vi "cw_2.vi"() -> ()   [LabVIEW 2022 SP3]
panel:
  out "sin(x)":dbl
  in  "dx":dbl
  out "Waveform Chart":dbl(graph)
  in  "stop":bool
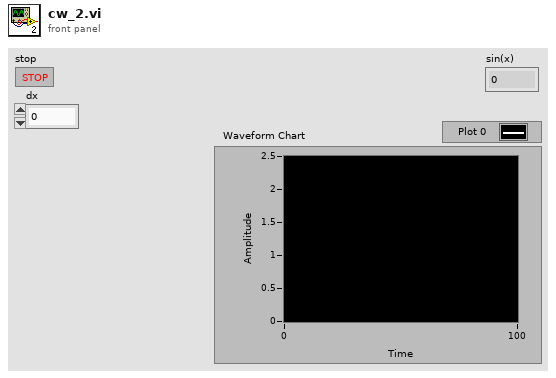
[diagram p1: front panel]
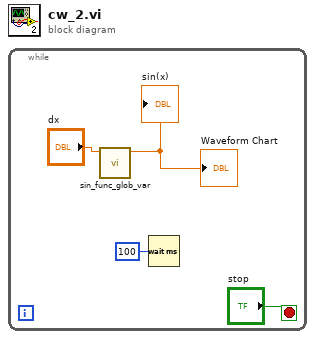
[diagram p0: block diagram]
diagram:
  n1 = while {
    stop <- "stop" stop-if-true
    n2 = call "sin_func_glob_var.vi"("dx"="dx") -> ("sin x"=→"Waveform Chart" →"sin(x)":dbl)  [unwired: 9 in, 1 out]
    n3 = Wait (ms)(milliseconds to wait=u32 100) -> ()  [unwired: 1 out]
  }
